vi "Convert_Sec_2_Date.vi"() -> ()   [LabVIEW 2020]
panel:
  out "time string":string
  out "date string":string
  in  "Numeric":dbl format="%#.0f"
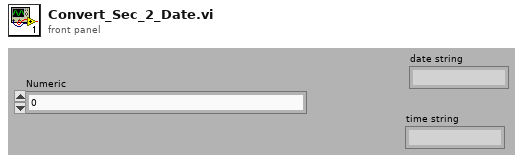
[diagram p1: front panel]
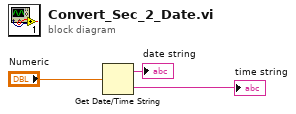
[diagram p0: block diagram]
diagram:
  n1 = Get Date/Time String(seconds (now)="Numeric") -> (date string=→"date string":string, time string=→"time string":string)  [unwired: 2 out]
